vi "Check Shutdown.vi"(8 "error in (no error)":errorcluster, 11 "Level Meter in":refnum<class "Level Meter.lvclass">) -> (0 "error out":errorcluster, 2 "Shut down":bool, 3 "Level Meter out":refnum<class "Level Meter.lvclass">)   [LabVIEW 2012, in "Level Meter.lvclass"]
uses:
  Level Meter.lvclass
  Level Meter.lvclass/Level Meter.ctl
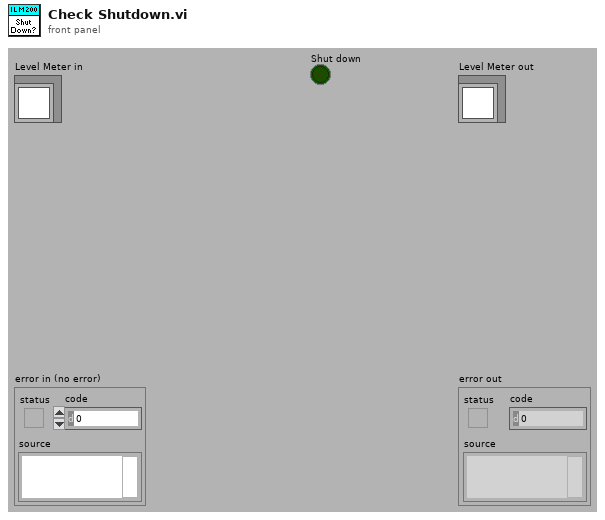
[diagram p1: front panel]
types:
  T1 = typedef "OxfordAddress.ctl" = cluster{"Com Port":i32, "ISOBUS Address":i32, "GPIB Address":i16, "Communication":enum16{"RS232", "ISOBUS", "GPIB", "Gateway"}}
  T2 = typedef "ILMRelayStatus.ctl" = cluster{"Shut down":bool, "Alarm sound":bool, "Alarm state":bool, "Silence prohib":bool, "Relay1 active":bool, "Relay 2 active":bool, "Relay 3 active":bool, "Relay 4 active":bool}
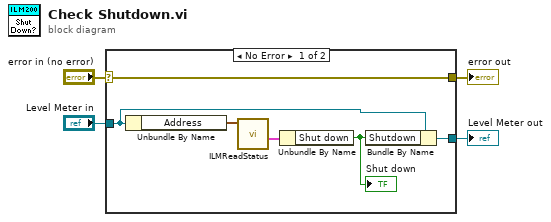
[diagram p0: block diagram]
diagram:
  n1 = case shown="No Error" "error in (no error)" {
    selector: "error in (no error)" -> [w10 w12]
    tunnel: [w10 w12] -> w3
    tunnel: [w8 w11] -> w1
    tunnel: "Level Meter in" -> [w6 w11]
    frame No Error {
      n2 = Unbundle By Name(w6) -> ("Address"=w5:T1)
      n3 = call "ILMReadStatus.vi"("Instrument address"=w5) -> ("Relay"=w9:T2)  [unwired: 6 out]
      n4 = Unbundle By Name(w9) -> ("Shut down"=w7:bool)
      "Shut down" <- w7
      n5 = Bundle By Name(cluster=w6, "Shutdown"=w7) -> (w8:refnum<class "Level Meter.lvclass">)
    }
    frame Error {
    }
  }
  "error out" <- w3
  "Level Meter out" <- w1
